vi "Write SyncDevice.vi"(10 "SyncDevice":bool, 11 "Template in":refnum<class "Template.lvclass">) -> (3 "Template out":refnum<class "Template.lvclass">)   [LabVIEW 2020, in "Template.lvlib" / "Template.lvclass"]
uses:
  Template.lvclass
  Template.lvclass/Template.ctl
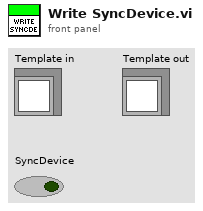
[diagram p1: front panel]
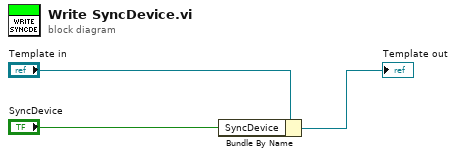
[diagram p0: block diagram]
diagram:
  n1 = Bundle By Name(cluster="Template in", "SyncDevice"="SyncDevice") -> (→"Template out":refnum<class "Template.lvclass">)
